vi "Camera Servo PID.vi"(1 "Front Camera In":T1) -> (0 "Front Camera Out":T1)   [LabVIEW 2013]
uses:
  <vilib>/addons/control/pid/pid.llb/PID Control Input Filter (DBL).vi
  <vilib>/addons/control/pid/NI_PID_pid.lvlib
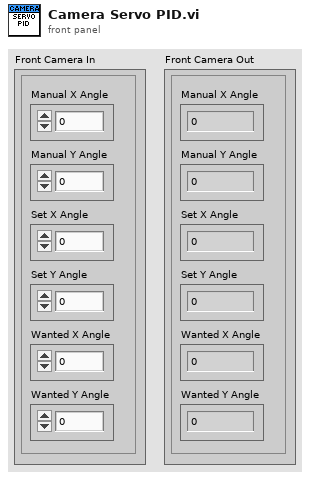
[diagram p1: front panel]
types:
  T1 = cluster{"Manual X Angle":dbl, "Manual Y Angle ":dbl, "Set X Angle":dbl, "Set Y Angle ":dbl, "Wanted X Angle":dbl, "Wanted Y Angle  ":dbl}
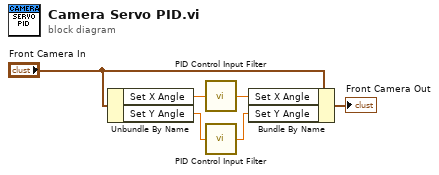
[diagram p0: block diagram]
diagram:
  n1 = Unbundle By Name("Front Camera In") -> ("Set X Angle"=w4:dbl, "Set Y Angle"=w3:dbl)
  n2 = call-poly <vilib>:"PID Control Input Filter.vi"("input"=w4) -> ("output"=w6:dbl)  [unwired: 1 in, 3 out]
  n3 = call-poly <vilib>:"PID Control Input Filter.vi"("input"=w3) -> ("output"=w5:dbl)  [unwired: 1 in, 3 out]
  n4 = Bundle By Name(cluster="Front Camera In", "Set X Angle"=w6, "Set Y Angle"=w5) -> (→"Front Camera Out":T1)
